vi "Error Strings.vi"() -> ()   [LabVIEW 2019, in "SEECD Shared.lvlib"]
uses:
  SEECD Shared.lvlib
panel:
  in  "Tab Control":enum32{"Legacy", "Reserved Range"}(tab)=enum."Reserved Range"
  out "537700":string="EtherCAT master %d not found."
  out "537701":string="EtherCAT slave %d not found."
  out "537702":string="Module \"%s\" (slot %d) not found."
  out "537703":string="Asynchronous loop in unexpected state."
  out "537704":string="Timeout communicating with asyncronyous loop."
  out "537705":string="UDV \"%s\" not found."
  out "537706":string="The EtherCAT slave \"%s\" configuration does not match the currently deployed FPGA personality."
  out "537707":string="UDV container not found."
  out "537710":string="Unsupported file type.  Please select a valid .lvbitx file."
  out "537711":string="Unsupported module type. This module is not supported in this version of VeriStand."
  out "537713":string="ECAT Slave I/O Variable \"%s\" does not match configuration to SDF \"%s\"."
  out "537714":string="Timeout communicating with EtherCAT reconfiguration loop."
  out "-732172":string
  out "-732171":string
  out "-732173":string
  out "-732174":string
  out "-732170":string
  out "-732167":string
  out "-732166":string
  out "-732168":string
  out "-732169":string
  out "-732165":string
  out "-732162":string
  out "-732161":string
  out "-732163":string
  out "-732164":string
  out "-732160":string
  out "-732157":string
  out "-732156":string
  out "-732158":string
  out "-732159":string
  out "-732152":string="The reference ID provided does not match the expected GUID, \"%s\", or cannot be found."
  out "-732151":string="The reference ID provided does not match the expected name, \"%s\", or cannot be found."
  out "-732150":string="The Scan Engine and EtherCAT custom device already exists."
  out "-732153":string="The Local Chassis already exists."
  out "-732154":string="An insufficient number of channels was provided for module creation."
  out "-732155":string="This module and/or mode is not currently supported by the API."
  # "These error codes are in a user-defined range, and are not being migrated to the range reserved for the Scan Engine EtherCAT custom device due to compatibility concerns.\n\nNo new error codes should be added to this range."
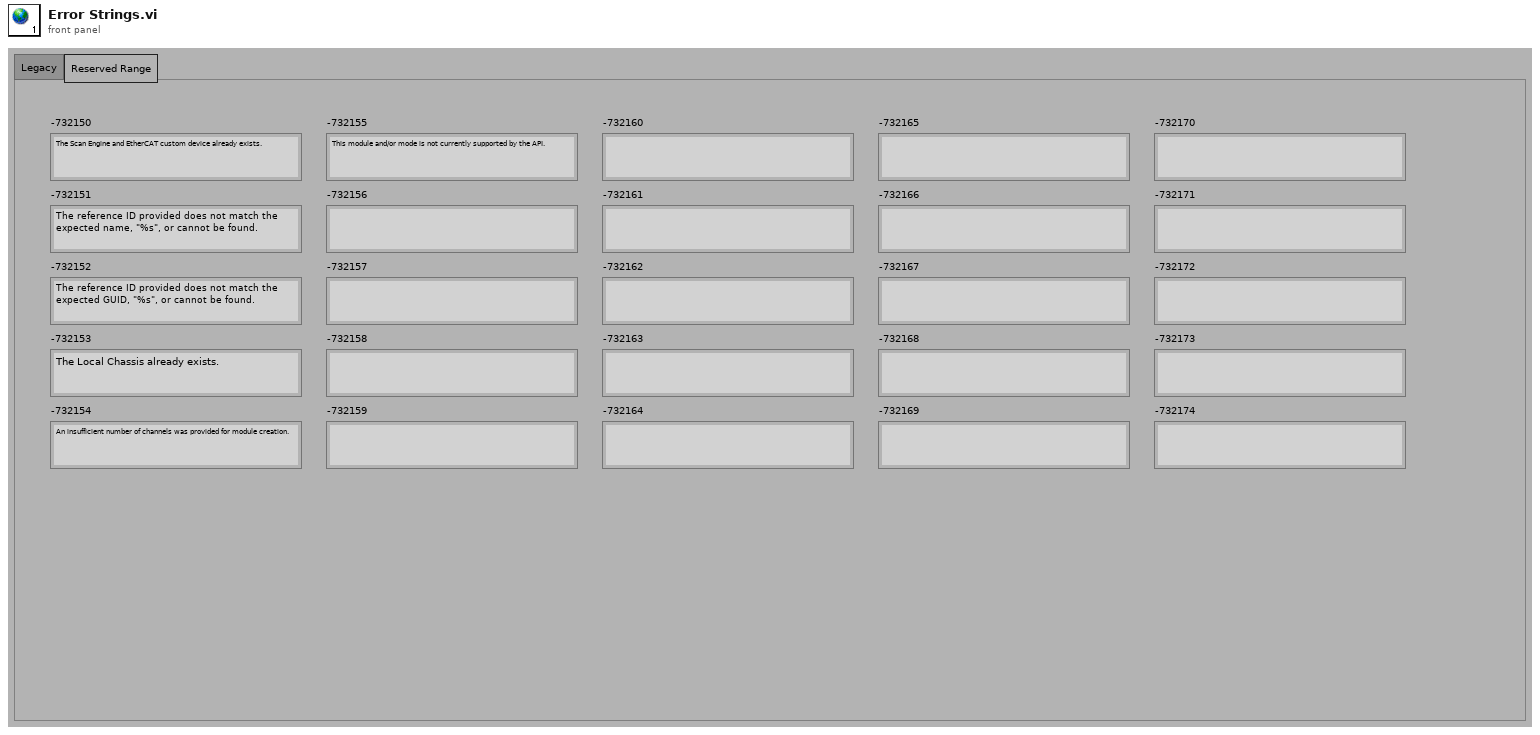
[diagram p1: front panel]
diagram:
